vi "List Top Level VIs__ogtk.vi"(8 "error in (no error)":errorcluster, 11 "LLB Path":path) -> (0 "error out":errorcluster, 2 "Top-Level VIs":string[](array[string]), 3 "dup LLB Path":path)   [LabVIEW 2018]
doc: "Lists the Top-Level VIs in an LLB or EXE."
uses:
  <userlib>/_OpenG.lib/array/array.llb/Conditional Auto-Indexing Tunnel (String)__ogtk.vi
panel:
  # "List Top Level VIs.vi\n\nLists the Top-Level VIs in an LLB\n\nPlease visit http://www.OpenG.org to learn about the\nOpen Source LabVIEW software movement.\n\nNOTICE -- YOU MUST LEAVE THIS NOTICE IN PLACE.  PER THE TERMS OF THE LICENSE BELOW, YOU MAY SUBLICENSE THIS SOFTWARE \nIN ANY WAY THAT DOES NOT CONFLICT WITH THIS LICENSE.\n\n### BSD License (http://www.opensource.org/licenses/bsd-license.php) Begin ###\n \nCopyright (c) 2002, Jim Kring <jim@jimkring.com>\n\nAll rights reserved.\n\nRedistribution and use in source and binary forms, with or without modification, are permitted provided that the following conditions are met:\n\n    * Redistributions of source code must retain the above copyright notice, this list of conditions and the following disclaimer.\n    * Redistributions in binary form must reproduce the above copyright notice, this list of conditions and the following disclaimer in the \n       documentation and/or other materials provided with the distribution.\n    * Neither the name of SciWare, James Kring, Inc., nor the names of its contributors may be used to endorse or promote products derived \n       from this software without specific prior written permission.\n\nTHIS SOFTWARE IS PROVIDED BY THE COPYRIGHT HOLDERS AND CONTRIBUTORS \"AS IS\" AND ANY EXPRESS OR IMPLIED WARRANTIES, \nINCLUDING, BUT NOT LIMITED TO, THE IMPLIED WARRANTIES OF MERCHANTABILITY AND FITNESS FOR A PARTICULAR PURPOSE ARE \nDISCLAIMED. IN NO EVENT SHALL THE COPYRIGHT OWNER OR CONTRIBUTORS BE LIABLE FOR ANY DIRECT, INDIRECT, INCIDENTAL,\n SPECIAL, EXEMPLARY, OR CONSEQUENTIAL DAMAGES (INCLUDING, BUT NOT LIMITED TO, PROCUREMENT OF SUBSTITUTE GOODS OR \nSERVICES; LOSS OF USE, DATA, OR PROFITS; OR BUSINESS INTERRUPTION) HOWEVER CAUSED AND ON ANY THEORY OF LIABILITY, \nWHETHER IN CONTRACT, STRICT LIABILITY, OR TORT (INCLUDING NEGLIGENCE OR OTHERWISE) ARISING IN ANY WAY OUT OF THE USE \nOF THIS SOFTWARE, EVEN IF ADVISED OF THE POSSIBILITY OF SUCH DAMAGE.\n\n### BSD License End ###"
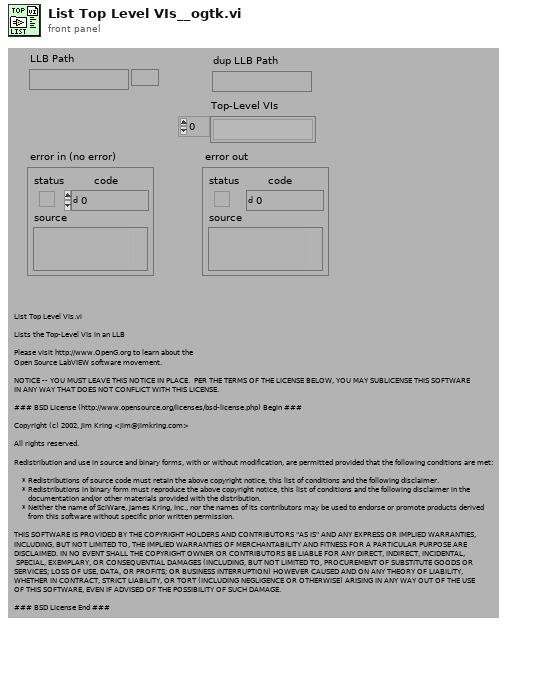
[diagram p1: front panel]
types:
  T1 = typedef "Librarian File Info Out.ctl" = cluster{"creation date":u32, "last mod date":u32, "type":string, "creator":string, "LV version":i32, "size":i32, "top level":bool}
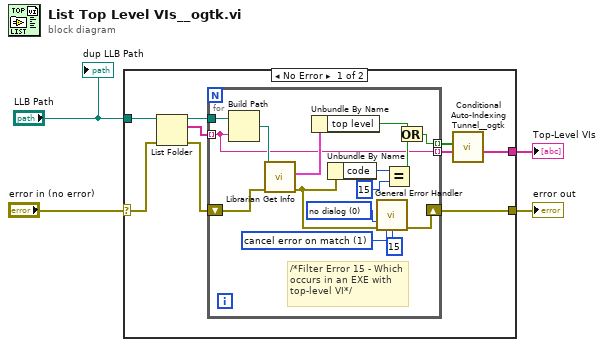
[diagram p0: block diagram]
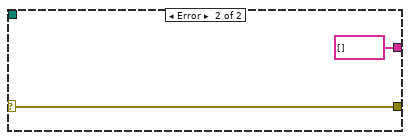
[diagram p2: hidden frame]
diagram:
  n1 = case shown="No Error" "error in (no error)" {
    selector: "error in (no error)" -> [w5 w29]
    tunnel: [w9 string[] [] ("Filtered Array out")] -> w4
    tunnel: [w8 w29] -> w3
    tunnel: "LLB Path" -> [w6 _]
    frame No Error {
      n2 = List Folder(path=w6, error in=w5) -> (path out=w13:path, filenames=w12:string[], error out=w7:errorcluster)  [unwired: 2 in, 1 out]
      n3 = for {
        tunnel: w13 -> [w28]
        tunnel: w12 -> [w19] mode=indexing
        shift-right: [w14] -> w8
        shift-left: w7 -> [w26]
        tunnel: [w22] -> w10 mode=indexing
        tunnel: [w19] -> w11 mode=indexing
        w15 = 1 items=["no exception", "cancel error on match", "set error on match"] ("[exception action] (none:0)")
        w16 = u16 0 items=["no dialog", "OK message", "continue or stop message"] ("type of dialog (OK msg:1)")
        # "/*Filter Error 15 - Which occurs in an EXE with top-level VI*/"
        n4 = Build Path(base path=w28, name or relative path=w19) -> (appended path=w27:path)
        n5 = call <vilib>:"Librarian Get Info.vi"("error in (no error)"=w26, "path"=w27) -> ("error out"=w18:errorcluster, "file information"=w25:T1)  [unwired: 7 in, 1 out]
        n6 = Unbundle By Name(w25) -> ("top level"=w20:bool)
        n7 = Unbundle By Name(w18) -> ("code"=w24:i32)
        n8 = call <vilib>:"General Error Handler.vi"("type of dialog (OK msg:1)"=w16, "error in (no error)"=w18, "[exception action] (none:0)"=w15, "[exception code]"=15) -> ("error out"=w14:errorcluster)  [unwired: 7 in, 4 out]
        n9 = Equal?(x=w24, y=15) -> (x = y?=w21:bool)
        n10 = Or(x=w20, y=w21) -> (x .or. y?=w22:bool)
      }
      n11 = call-poly <userlib>:"Conditional Auto-Indexing Tunnel__ogtk.vi"("Array in"=w11, "Elements to keep"=w10) -> ("Filtered Array out"=w9:string[])  [unwired: 5 in]
    }
    frame Error {
    }
  }
  "error out" <- w3
  "Top-Level VIs" <- w4
  "dup LLB Path" <- "LLB Path"
